vi "Get Limit Test Lower Limit.vi"(0 "VISA resource name":refnum<visa-resource-name>, 5 "Limit Test Number (2)":u16=2 min=1 max=2 step=1, 7 "Function (0: Volts)":u16(ring) items=["Volts", "Current", "Resistance", "Digitize Voltage", "Digitize Current"], 11 "error in (no error)":errorcluster) -> (4 "VISA resource name out":refnum<visa-resource-name>, 6 "Lower Limit":dbl, 15 "error out":errorcluster)   [LabVIEW 2017, in "Keithley 2450.lvlib"]
doc: "This VI returns the lower limit for limit tests."
uses:
  Keithley 2450.lvlib
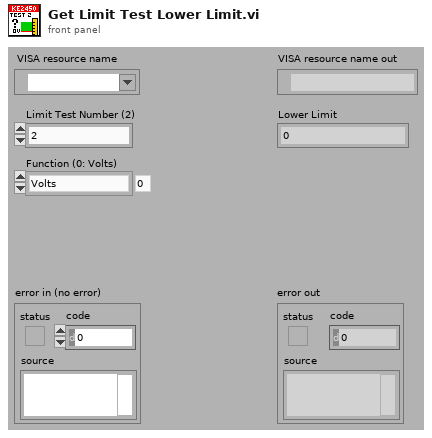
[diagram p1: front panel]
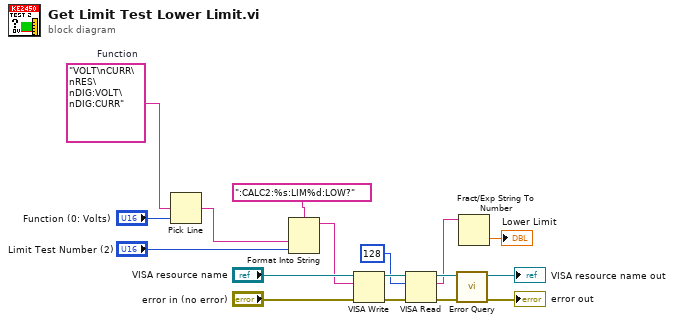
[diagram p0: block diagram]
diagram:
  w11 = "VOLT\nCURR\nRES\nDIG:VOLT\nDIG:CURR"  # Function
  n1 = Pick Line(multi-line string=w11, line index="Function (0: Volts)") -> (output string=w9:string)  [unwired: 1 out]
  n2 = Format Into String(format string=":CALC2:%s:LIM%d:LOW?", w9, "Limit Test Number (2)") -> (resulting string=w12:string)  [unwired: 2 in, 1 out]
  n3 = VISA Write(VISA resource name="VISA resource name", write buffer=w12, error in (no error)="error in (no error)") -> (VISA resource name out=w5:refnum<visa-resource-name>, error out=w7:errorcluster)  [unwired: 1 out]
  n4 = VISA Read(VISA resource name=w5, byte count=u32 128, error in (no error)=w7) -> (VISA resource name out=w4:refnum<visa-resource-name>, read buffer=w2:string, error out=w6:errorcluster)  [unwired: 1 out]
  n5 = call "Error Query.vi"("error in (no error)"=w6, "VISA resource name"=w4) -> ("error out"=→"error out":errorcluster, "VISA resource name out"=→"VISA resource name out":refnum<visa-resource-name>)  [unwired: 8 out]
  n6 = Fract/Exp String To Number(string=w2) -> (number=→"Lower Limit":dbl)  [unwired: 3 in, 1 out]
